vi "Measurement Setting.vi"(7 "Measurement Type (0:Impedance)":u32(ring) items=["Impedance ", "Gain - Phase", "Impedance With Probe"], 8 "error in (no error)":errorcluster, 9 "Gain-Phase (0:Tch/Rch [dB] - Theta)":u32(ring) items=["Tch/Rch [dB] - Theta", "Tch/Rch - theta", "Tch/Rch [dB] - tau", "Tch-Rch [V]", "Tch-Rch [dBm]", "Tch-Rch [dBV]"], 10 "Impedance (0:| Z | - Theta )":u32(ring) items=["| Z | -Ttheta ", "R - X", "Ls-Rs", "Ls-Q", "Cs-Rs", "Cs-Q", "Cs-D", "|Y|-Theta", "G-B", "Lp-G", "Lp-Q", "Cp-G", "Cp-Q", "Cp-D", "|Z|-Ls", "|Z|-Cs", "|Z|-Lp", "|Z|-Cp", "Lp-Rp", "Cp-Rp"], 11 "VISA resource name":refnum<visa-resource-name>) -> (0 "error out":errorcluster, 3 "VISA resource name out":refnum<visa-resource-name>)   [LabVIEW 2011, in "Agilent 4194.lvlib"]
doc: "This function sets the type of impedance or gain-phase measurement."
uses:
  <instrlib>/Agilent 4194/Agilent 4194.lvlib
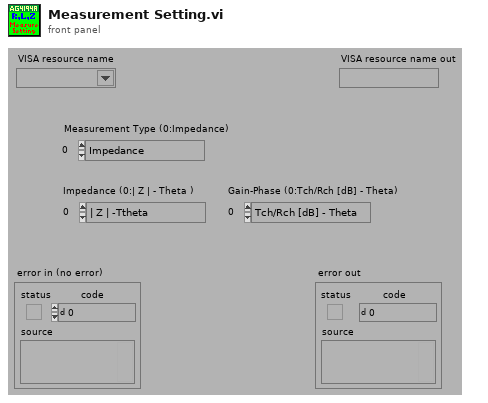
[diagram p1: front panel]
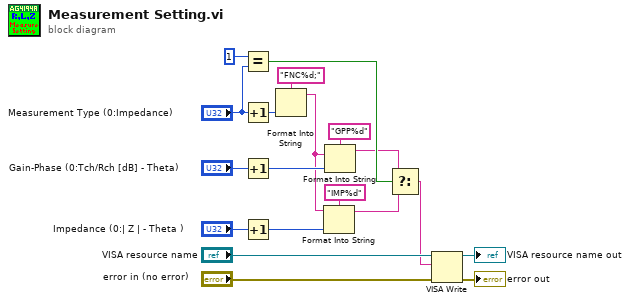
[diagram p0: block diagram]
diagram:
  n1 = Equal?(x=u32 1 ("y"), y="Measurement Type (0:Impedance)") -> (x = y?=w7:bool)
  n2 = Increment(x="Measurement Type (0:Impedance)") -> (x+1=w14:u32)
  n3 = Increment(x="Gain-Phase (0:Tch/Rch [dB] - Theta)") -> (x+1=w12:u32)
  n4 = Increment(x="Impedance (0:| Z | - Theta )") -> (x+1=w9:u32)
  n5 = Format Into String(format string="FNC%d;", w14) -> (resulting string=w6:string)  [unwired: 2 in, 1 out]
  n6 = Format Into String(format string="IMP%d", initial string=w6, w9) -> (resulting string=w1:string)  [unwired: 1 in, 1 out]
  n7 = Format Into String(format string="GPP%d", initial string=w6, w12) -> (resulting string=w2:string)  [unwired: 1 in, 1 out]
  n8 = Select(t=w2, s=w7, f=w1) -> (s? t:f=w5:string)
  n9 = VISA Write(VISA resource name="VISA resource name", write buffer=w5, error in (no error)="error in (no error)") -> (VISA resource name out=→"VISA resource name out":refnum<visa-resource-name>, error out=→"error out":errorcluster)  [unwired: 1 out]
